vi "Center on Trigger.vi"(8 "Threshold":dbl, 9 "Center":bool, 10 "Array":dbl[](array[numeric])) -> (1 "XScale Fit":i32=2, 2 "Max":dbl, 3 "Min":dbl)   [LabVIEW 2012]
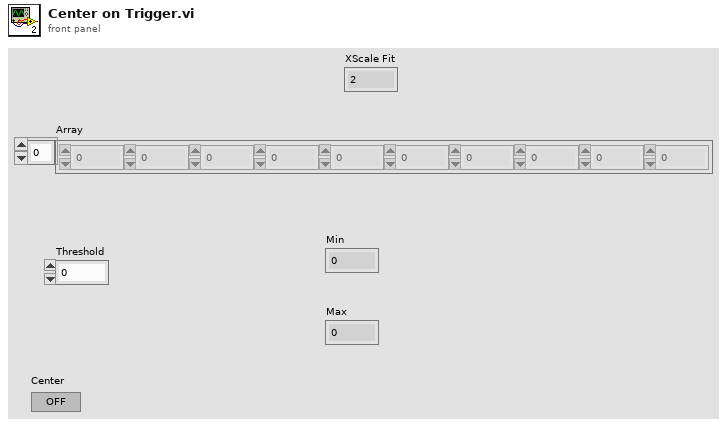
[diagram p1: front panel]
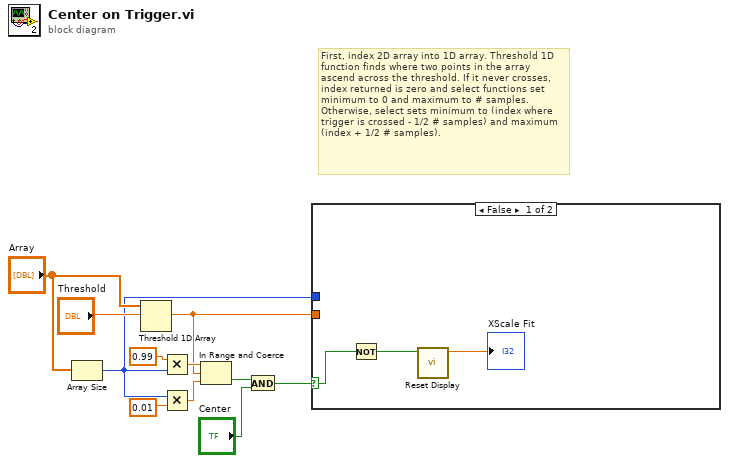
[diagram p0: block diagram]
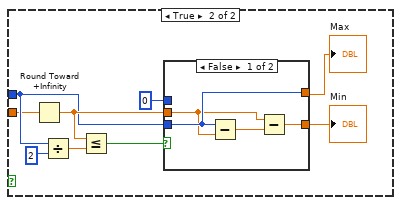
[diagram p2: hidden frame]
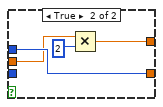
[diagram p3: hidden frame]
diagram:
  # "First, index 2D array into 1D array. Threshold 1D function finds where two points in the array  ascend across the threshold. If it never crosses, index returned is zero and select functions set minimum to 0 and maximum to # samples. Otherwise, select sets minimum to (index where trigger is crossed - 1/2 # samples) and maximum (index + 1/2 # samples)."
  n1 = Array Size(array="Array") -> (size(s)=w3:i32)
  n2 = Threshold 1D Array(2:"Threshold", 3:"Array") -> (0:w2:dbl)  [unwired: 1 in]
  n3 = Multiply(x=0.99, y=w3) -> (x*y=w4:dbl)
  n4 = Multiply(x=w3, y=0.01) -> (x*y=w6:dbl)
  n5 = In Range and Coerce(upper limit=w4, x=w2, lower limit=w6) -> (In Range?=w9:bool)  [unwired: 1 out]
  n6 = And(x=w9, y="Center") -> (x .and. y?=w1:bool)
  n7 = case shown="False" w1 {
    selector: w1 -> [w14 _]
    tunnel: w3 -> [_ w16]
    tunnel: w2 -> [_ w15]
    frame False {
      n8 = Not(x=w14) -> (.not. x?=w13:bool)
      n9 = call "Reset Display.vi"("Reset Button"=w13) -> ("XScale Fit"=→"XScale Fit":dbl)  [unwired: 9 in, 1 out]
    }
    frame True {
      n10 = Round Toward +Infinity(x=w15) -> (ceil(x): smallest int >= x=w19:dbl)
      n11 = Divide(x=w16, y=2) -> (x/y=w22:dbl)
      n12 = Less Or Equal?(x=w19, y=w22) -> (x <= y?=w20:bool)
      n13 = case shown="False" w20 {
        tunnel: 0 -> [_ w29]
        tunnel: w16 -> [w27 _]
        tunnel: [w27 w30] -> w18
        tunnel: [w24 w29] -> w17
        tunnel: w19 -> [w26 w28]
        frame False {
          n14 = Subtract(x=w27, y=w26) -> (x-y=w25:dbl)
          n15 = Subtract(x=w26, y=w25) -> (x-y=w24:dbl)
        }
        frame True {
          n16 = Multiply(x=w28, y=2) -> (x*y=w30:dbl)
        }
      }
      "Max" <- w18
      "Min" <- w17
    }
  }
